vi "Initialization VI.vi"(8 "error in (no error)":errorcluster, 10 "Custom XML":string, 11 "Device Item Ref in":T1 format="%.0x") -> (0 "error out":errorcluster, 3 "Device Item Ref out":T1 format="%.0x")   [LabVIEW 2020, in "Waveform Analog Output System Explorer.lvlib"]
uses:
  Waveform Analog Output System Explorer.lvlib
  <vilib>/NI VeriStand/Custom Device API/Custom Device Item Ref.ctl
  <vilib>/NI VeriStand/Custom Device API/Custom Device Channel.ctl
  <vilib>/NI VeriStand/Custom Device API/Custom Device Channel Type.ctl
  Number of AO Channels.ctl
  <vilib>/NI VeriStand/Custom Device API/Custom Device Loop Type.ctl
  <vilib>/NI VeriStand/Custom Device API/Custom Device Timed Loop Priority.ctl
  Shared/Constants.vi
  <vilib>/NI VeriStand/Custom Device API/Set Item Property (Variant).vi
  <vilib>/NI VeriStand/Custom Device API/Set Item Property (U16).vi
  <vilib>/NI VeriStand/Custom Device API/Custom Device API.lvlib
  Shared/Waveform Analog Output Shared.lvlib
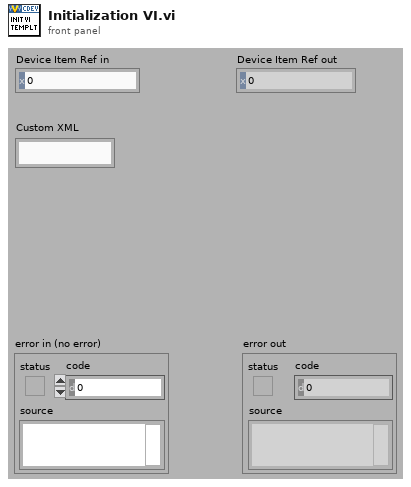
[diagram p1: front panel]
types:
  T1 = typedef "Custom Device API.lvlib/Custom Device Item Ref.ctl" = u64
  T2 = typedef "Custom Device API.lvlib/Custom Device Timed Loop Priority.ctl" = enum32{"Low", "Medium", "High"}
  T3 = typedef "Custom Device API.lvlib/Custom Device Loop Type.ctl" = enum32{"While Loop", "Timed Loop"}
  T4 = typedef "Custom Device API.lvlib/Custom Device Channel.ctl" = cluster{"Type":T5, "Units":string, "Default Value":dbl, "Faultable":bool, "Scalable":bool}
  T5 = typedef "Custom Device API.lvlib/Custom Device Channel Type.ctl" = enum16{"Input", "Output"}
  T6 = typedef "Waveform Analog Output System Explorer.lvlib/Number of AO Channels.ctl" = u16
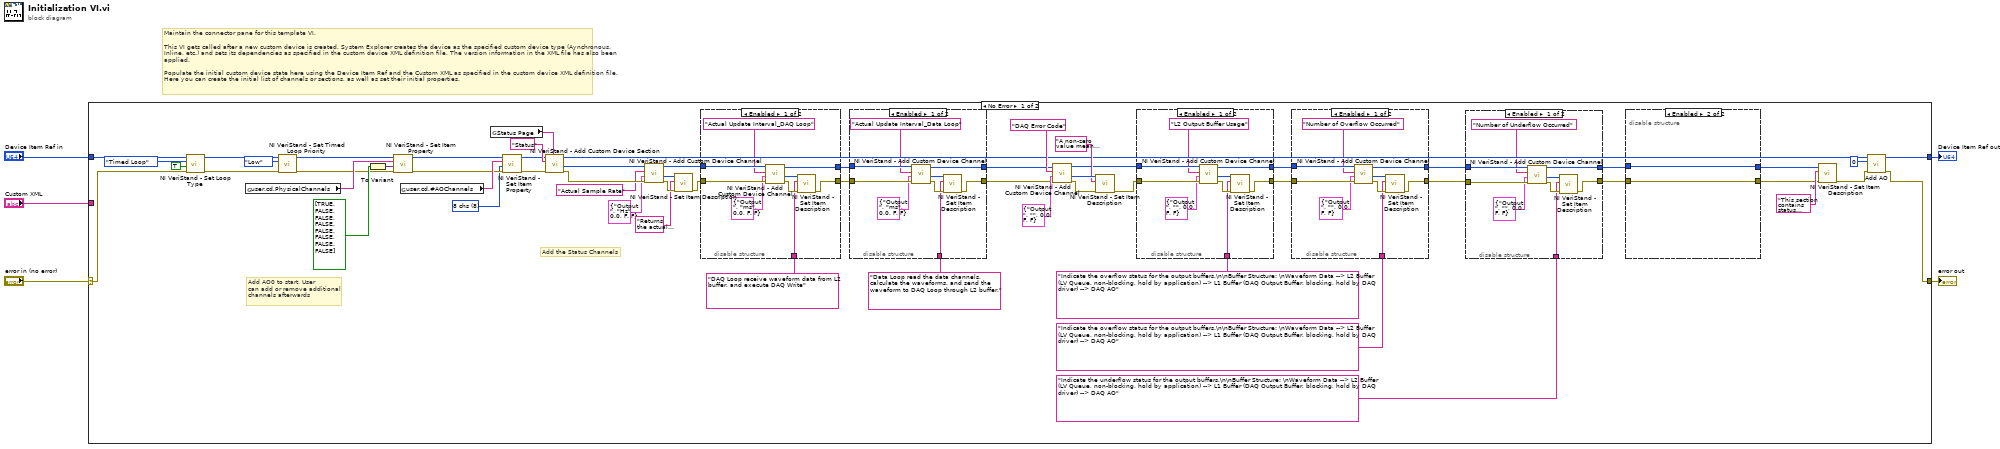
[diagram p0: block diagram]
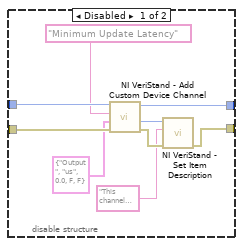
[diagram p7: hidden frame]
diagram:
  # "Maintain the connector pane for this template VI.\n\nThis VI gets called after a new custom device is created. System Explorer creates the device as the specified custom device type (Aynchronous, Inline, etc.) and sets its dependencies as specified in the custom device XML definition file. The version information in the XML file has also been applied.\n\nPopulate the initial custom device state here using the Device Item Ref and the Custom XML as specified in the custom device XML definition file. Here you can create the initial list of channels or sections, as well as set their initial properties."
  n1 = case shown="No Error" "error in (no error)" {
    selector: "error in (no error)" -> [w26 w132]
    tunnel: [w34 w132] -> w5
    tunnel: [w35 w131] -> w3
    tunnel: "Device Item Ref in" -> [w64 w131]
    tunnel: "Custom XML" -> [_ _]
    frame No Error {
      w38 = T6 8 items=["2 chs"=2, "4 chs"=4, "8 chs"=8, "32 chs"=32, "64 chs"=64] ("Number of AO Channels")
      # "Add the Status Channels"
      # "Add AO0 to start. User\ncan add or remove additional\nchannels afterwards"
      n2 = call <vilib>:"NI VeriStand - Set Loop Type.vi"("error in (no error)"=w26, "Use Device Clock (Timed Loops only)"=TRUE, "Loop type"=Custom_Device_Loop_Type."Timed Loop", "Device Ref in"=w64) -> ("error out"=w27:errorcluster, "Device Ref out"=w32:T1)  [unwired: 6 in]
      n3 = global read "Constants.vi" "user.cd.PhysicalChannels"() -> (w58:string)
      n4 = call <vilib>:"NI VeriStand - Set Timed Loop Priority.vi"("error in (no error)"=w27, "Priority"=Custom_Device_Timed_Loop_Priority."Low", "Device Ref in"=w32) -> ("error out"=w25:errorcluster, "Device Ref out"=w30:T1)  [unwired: 7 in]
      n5 = To Variant(anything=bool[] [TRUE, FALSE, FALSE, FALSE, FALSE, FALSE, FALSE, FALSE]) -> (Variant=w57:variant)
      n6 = call-poly <vilib>:"NI VeriStand - Set Item Property.vi"("error in (no error)"=w25, "Value"=w57, "Property Name"=w58, "Item Ref in"=w30) -> ("error out"=w40:errorcluster, "Item Ref out"=w42:T1)  [unwired: 5 in, 1 out]
      n7 = global read "Constants.vi" "user.cd.#AOChannels"() -> (w43:string)
      n8 = global read "Constants.vi" "Status Page"() -> (w46:string)
      n9 = call-poly <vilib>:"NI VeriStand - Set Item Property.vi"("error in (no error)"=w40, "Value"=w38, "Property Name"=w43, "Item Ref in"=w42) -> ("error out"=w39:errorcluster, "Item Ref out"=w41:T1)  [unwired: 5 in, 1 out]
      n10 = call <vilib>:"NI VeriStand - Add Custom Device Section.vi"("GUID (Default Section)"=w46, "error in (no error)"=w39, "Section Name"="Status", "Parent Ref in"=w41) -> ("error out"=w61:errorcluster, "Section Ptr"=w62:T1, "Parent Ref out"=w36:T1)  [unwired: 4 in, 1 out]
      n11 = call <vilib>:"NI VeriStand - Add Custom Device Channel.vi"("error in (no error)"=w61, "Channel"=T4 {"Type"=enum."Output", "Units"="Hz", "Default Value"=0.0, "Faultable"=FALSE, "Scalable"=FALSE}, "Channel Name"="Actual Sample Rate", "Parent Ref in"=w62) -> ("error out"=w49:errorcluster, "Channel Ref"=w50:T1, "Parent Ref out"=w24:T1)  [unwired: 4 in, 1 out]
      n12 = call <vilib>:"NI VeriStand - Set Item Description.vi"("error in (no error)"=w49, "Description"="Returns the actual sample rate that the DAQ card is using to generate the waveforms. This value is returned during initialization and will not change as the system runs.", "Item Ref in"=w50) -> ("error out"=w22:errorcluster)  [unwired: 6 in, 2 out]
      n13 = disable-structure shown="Enabled" {
        disable-tunnel: w24 -> [w106 w108]
        disable-tunnel: w22 -> [w105 w107]
        disable-tunnel: [w100 w108] -> w23
        disable-tunnel: [w99 w107] -> w21
        disable-tunnel: "DAQ Loop receive waveform data from L2 buffer, and execute DAQ Write" ("Description") -> [w98 _]
        frame Enabled {
          n14 = call <vilib>:"NI VeriStand - Add Custom Device Channel.vi"("error in (no error)"=w105, "Channel"=T4 {"Type"=enum."Output", "Units"="ms", "Default Value"=0.0, "Faultable"=FALSE, "Scalable"=FALSE}, "Channel Name"="Actual Update Interval_DAQ Loop", "Parent Ref in"=w106) -> ("error out"=w101:errorcluster, "Channel Ref"=w102:T1, "Parent Ref out"=w100:T1)  [unwired: 4 in, 1 out]
          n15 = call <vilib>:"NI VeriStand - Set Item Description.vi"("error in (no error)"=w101, "Description"=w98, "Item Ref in"=w102) -> ("error out"=w99:errorcluster)  [unwired: 6 in, 2 out]
        }
        frame Disabled {
        }
      }
      n16 = disable-structure shown="Enabled" {
        disable-tunnel: w23 -> [w117 w119]
        disable-tunnel: w21 -> [w116 w118]
        disable-tunnel: [w111 w119] -> w20
        disable-tunnel: [w110 w118] -> w19
        disable-tunnel: "Data Loop read the data channels, calculate the waveforms, and send the waveform to DAQ Loop through L2 buffer." ("Description") -> [w109 _]
        frame Enabled {
          n17 = call <vilib>:"NI VeriStand - Add Custom Device Channel.vi"("error in (no error)"=w116, "Channel"=T4 {"Type"=enum."Output", "Units"="ms", "Default Value"=0.0, "Faultable"=FALSE, "Scalable"=FALSE}, "Channel Name"="Actual Update Interval_Data Loop", "Parent Ref in"=w117) -> ("error out"=w112:errorcluster, "Channel Ref"=w113:T1, "Parent Ref out"=w111:T1)  [unwired: 4 in, 1 out]
          n18 = call <vilib>:"NI VeriStand - Set Item Description.vi"("error in (no error)"=w112, "Description"=w109, "Item Ref in"=w113) -> ("error out"=w110:errorcluster)  [unwired: 6 in, 2 out]
        }
        frame Disabled {
        }
      }
      n19 = call <vilib>:"NI VeriStand - Add Custom Device Channel.vi"("error in (no error)"=w19, "Channel"=T4 {"Type"=enum."Output", "Units"="", "Default Value"=0.0, "Faultable"=FALSE, "Scalable"=FALSE}, "Channel Name"="DAQ Error Code", "Parent Ref in"=w20) -> ("error out"=w52:errorcluster, "Channel Ref"=w53:T1, "Parent Ref out"=w17:T1)  [unwired: 4 in, 1 out]
      n20 = call <vilib>:"NI VeriStand - Set Item Description.vi"("error in (no error)"=w52, "Description"="A non-zero value means an error has occurred and the custom device has shut down", "Item Ref in"=w53) -> ("error out"=w18:errorcluster)  [unwired: 6 in, 2 out]
      n21 = disable-structure shown="Enabled" {
        disable-tunnel: w17 -> [w84 w86]
        disable-tunnel: w18 -> [w83 w85]
        disable-tunnel: [w78 w86] -> w10
        disable-tunnel: [w77 w85] -> w9
        disable-tunnel: "Indicate the overflow status for the output buffers.\n\nBuffer Structure: \nWaveform Data --> L2 Buffer (LV Queue, non-blocking, hold by application) --> L1 Buffer (DAQ Output Buffer, blocking, hold by DAQ driver) --> DAQ AO" ("Description") -> [w76 _]
        frame Enabled {
          n22 = call <vilib>:"NI VeriStand - Add Custom Device Channel.vi"("error in (no error)"=w83, "Channel"=T4 {"Type"=enum."Output", "Units"="", "Default Value"=0.0, "Faultable"=FALSE, "Scalable"=FALSE}, "Channel Name"="L2 Output Buffer Usage", "Parent Ref in"=w84) -> ("error out"=w79:errorcluster, "Channel Ref"=w80:T1, "Parent Ref out"=w78:T1)  [unwired: 4 in, 1 out]
          n23 = call <vilib>:"NI VeriStand - Set Item Description.vi"("error in (no error)"=w79, "Description"=w76, "Item Ref in"=w80) -> ("error out"=w77:errorcluster)  [unwired: 6 in, 2 out]
        }
        frame Disabled {
        }
      }
      n24 = disable-structure shown="Enabled" {
        disable-tunnel: w10 -> [w73 w75]
        disable-tunnel: w9 -> [w72 w74]
        disable-tunnel: [w67 w75] -> w8
        disable-tunnel: [w66 w74] -> w7
        disable-tunnel: "Indicate the overflow status for the output buffers.\n\nBuffer Structure: \nWaveform Data --> L2 Buffer (LV Queue, non-blocking, hold by application) --> L1 Buffer (DAQ Output Buffer, blocking, hold by DAQ driver) --> DAQ AO" ("Description") -> [w65 _]
        frame Enabled {
          n25 = call <vilib>:"NI VeriStand - Add Custom Device Channel.vi"("error in (no error)"=w72, "Channel"=T4 {"Type"=enum."Output", "Units"="", "Default Value"=0.0, "Faultable"=FALSE, "Scalable"=FALSE}, "Channel Name"="Number of Overflow Occurred", "Parent Ref in"=w73) -> ("error out"=w68:errorcluster, "Channel Ref"=w69:T1, "Parent Ref out"=w67:T1)  [unwired: 4 in, 1 out]
          n26 = call <vilib>:"NI VeriStand - Set Item Description.vi"("error in (no error)"=w68, "Description"=w65, "Item Ref in"=w69) -> ("error out"=w66:errorcluster)  [unwired: 6 in, 2 out]
        }
        frame Disabled {
        }
      }
      n27 = disable-structure shown="Enabled" {
        disable-tunnel: w8 -> [w95 w97]
        disable-tunnel: w7 -> [w94 w96]
        disable-tunnel: [w89 w97] -> w16
        disable-tunnel: [w88 w96] -> w15
        disable-tunnel: "Indicate the underflow status for the output buffers.\n\nBuffer Structure: \nWaveform Data --> L2 Buffer (LV Queue, non-blocking, hold by application) --> L1 Buffer (DAQ Output Buffer, blocking, hold by DAQ driver) --> DAQ AO" ("Description") -> [w87 _]
        frame Enabled {
          n28 = call <vilib>:"NI VeriStand - Add Custom Device Channel.vi"("error in (no error)"=w94, "Channel"=T4 {"Type"=enum."Output", "Units"="", "Default Value"=0.0, "Faultable"=FALSE, "Scalable"=FALSE}, "Channel Name"="Number of Underflow Occurred", "Parent Ref in"=w95) -> ("error out"=w90:errorcluster, "Channel Ref"=w91:T1, "Parent Ref out"=w89:T1)  [unwired: 4 in, 1 out]
          n29 = call <vilib>:"NI VeriStand - Set Item Description.vi"("error in (no error)"=w90, "Description"=w87, "Item Ref in"=w91) -> ("error out"=w88:errorcluster)  [unwired: 6 in, 2 out]
        }
        frame Disabled {
        }
      }
      n30 = disable-structure shown="Enabled" {
        disable-tunnel: w16 -> [w128 w130]
        disable-tunnel: w15 -> [w127 w129]
        disable-tunnel: [w121 w130] -> w45
        disable-tunnel: [w120 w129] -> w44
        frame Disabled {
          n31 = call <vilib>:"NI VeriStand - Add Custom Device Channel.vi"("error in (no error)"=w127, "Channel"=T4 {"Type"=enum."Output", "Units"="us", "Default Value"=0.0, "Faultable"=FALSE, "Scalable"=FALSE}, "Channel Name"="Minimum Update Latency", "Parent Ref in"=w128) -> ("error out"=w123:errorcluster, "Channel Ref"=w124:T1, "Parent Ref out"=w121:T1)  [unwired: 4 in, 1 out]
          n32 = call <vilib>:"NI VeriStand - Set Item Description.vi"("error in (no error)"=w123, "Description"="This channel outputs the minimum latency expected for new parameter values to update the waveform. This latency is calculated based on the current write location in the output buffer when a parameter value change occurs. Note that the latency can be slightly higher based on write location of the HW buffer.", "Item Ref in"=w124) -> ("error out"=w120:errorcluster)  [unwired: 6 in, 2 out]
        }
        frame Enabled {
        }
      }
      n33 = call <vilib>:"NI VeriStand - Set Item Description.vi"("error in (no error)"=w44, "Description"="This section contains status channels useful for tracking the health of this custom device.", "Item Ref in"=w45) -> ("error out"=w33:errorcluster)  [unwired: 6 in, 2 out]
      n34 = call "Add AO.vi"("error in (no error)"=w33, "Physical Channel Number"=0, "Device Item Ref in"=w36) -> ("error out"=w34:errorcluster, "Parent Ref out"=w35:T1)  [unwired: 7 in]
    }
    frame Error {
    }
  }
  "error out" <- w5
  "Device Item Ref out" <- w3
